vi "Register Actor.vi"(8 "error in (no error)":errorcluster, 10 "CO2 Actor":refnum<class "CO2 Actor.lvclass">, 11 "cRIO-CO2 in":refnum<class "cRIO-CO2.lvclass">) -> (0 "error out":errorcluster, 3 "cRIO-CO2 out":refnum<class "cRIO-CO2.lvclass">)   [LabVIEW 2015, in "cRIO-Carbondioxide.lvlib" / "cRIO-CO2.lvlib" / "cRIO-CO2.lvclass"]
uses:
  cRIO-CO2.lvclass
  CO2 Actor/CO2 Actor.lvclass
  cRIO-CO2.lvclass/cRIO-CO2.ctl
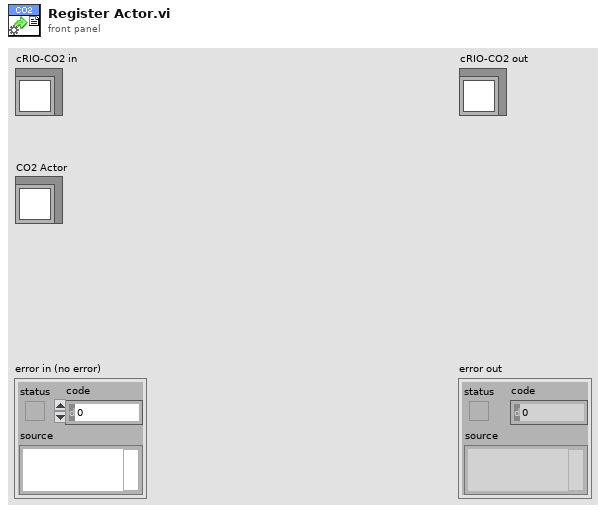
[diagram p1: front panel]
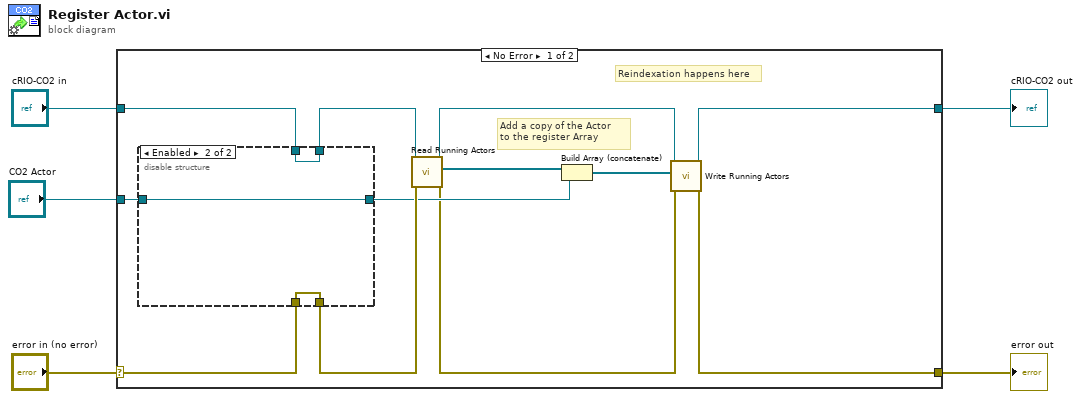
[diagram p0: block diagram]
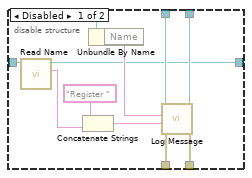
[diagram p2: hidden frame]
diagram:
  n1 = case shown="No Error" "error in (no error)" {
    selector: "error in (no error)" -> [w15 w32]
    tunnel: [w7 w32] -> w4
    tunnel: [w8 w31] -> w2
    tunnel: "cRIO-CO2 in" -> [w13 w31]
    tunnel: "CO2 Actor" -> [w14 _]
    frame No Error {
      # "Reindexation happens here"
      # "Add a copy of the Actor \nto the register Array"
      n2 = disable-structure shown="Enabled" {
        disable-tunnel: [w27 w30] -> w16
        disable-tunnel: w15 -> [w26 w29]
        disable-tunnel: w14 -> [w25 w28]
        disable-tunnel: w13 -> [w24 w30]
        disable-tunnel: [w19 w29] -> w12
        disable-tunnel: [w18 w28] -> w9
        frame Disabled {
          n3 = call "Read Name.vi"("CO2 Actor in"=w25) -> ("Name"=w23:string, "CO2 Actor out"=w18:refnum<class "CO2 Actor.lvclass">)  [unwired: 9 in]
          n4 = Concatenate Strings("Register " ("string"), w23) -> (w20:string)
          n5 = Unbundle By Name(w24) -> ("Name"=w21:string)
          n6 = call "Log Message.vi"("error in (no error)"=w26, "String"=w20, "Source Name"=w21, "cRIO-CO2 in"=w24) -> ("error out"=w19:errorcluster, "cRIO-CO2 out"=w27:refnum<class "cRIO-CO2.lvclass">)  [unwired: 6 in]
        }
        frame Enabled {
        }
      }
      n7 = call "Read Running Actors.vi"("error in (no error)"=w12, "cRIO-CO2 in"=w16) -> ("error out"=w6:errorcluster, "Running Actors"=w11:refnum<class "CO2 Actor.lvclass">[], "cRIO-CO2 out"=w17:refnum<class "cRIO-CO2.lvclass">)  [unwired: 7 in]
      n8 = Build Array (concatenate)(w11, w9) -> (w10:refnum<class "CO2 Actor.lvclass">[])
      n9 = call "Write Running Actors.vi"("error in (no error)"=w6, "Running Actors"=w10, "cRIO-CO2 in"=w17) -> ("error out"=w7:errorcluster, "cRIO-CO2 out"=w8:refnum<class "cRIO-CO2.lvclass">)  [unwired: 7 in]
    }
    frame Error {
    }
  }
  "error out" <- w4
  "cRIO-CO2 out" <- w2
